vi "Labial Pressure Marker.vi"(6 "Upper SPL":dbl, 8 "Error In":errorcluster, 9 "File Path":path, 10 "Pressure/Audio":dynamicdata(graph)) -> (0 "Error Out":errorcluster, 1 "File Path Indicator":path, 3 "Pressure Array":dbl[](array[numeric]))   [LabVIEW 2020, in "AnalysisSupport.lvlib"]
uses:
  AnalysisSupport.lvlib
  <vilib>/Utility/miscctls.llb/LVCursorListTypeDef.ctl
  <vilib>/Waveform/WDTOps.llb/WDT Get XY Value DBL.vi
panel:
  in  "Undo Button":bool
  out "Upper SPL Bound":dbl
  out "SPL":dbl
  out "Subset":dynamicdata(graph)
  out "Pressure":dynamicdata(graph)
  out "Interruptions Marked":i32
  out "Pressure":dbl
  in  "Done":bool
  in  "Add":bool
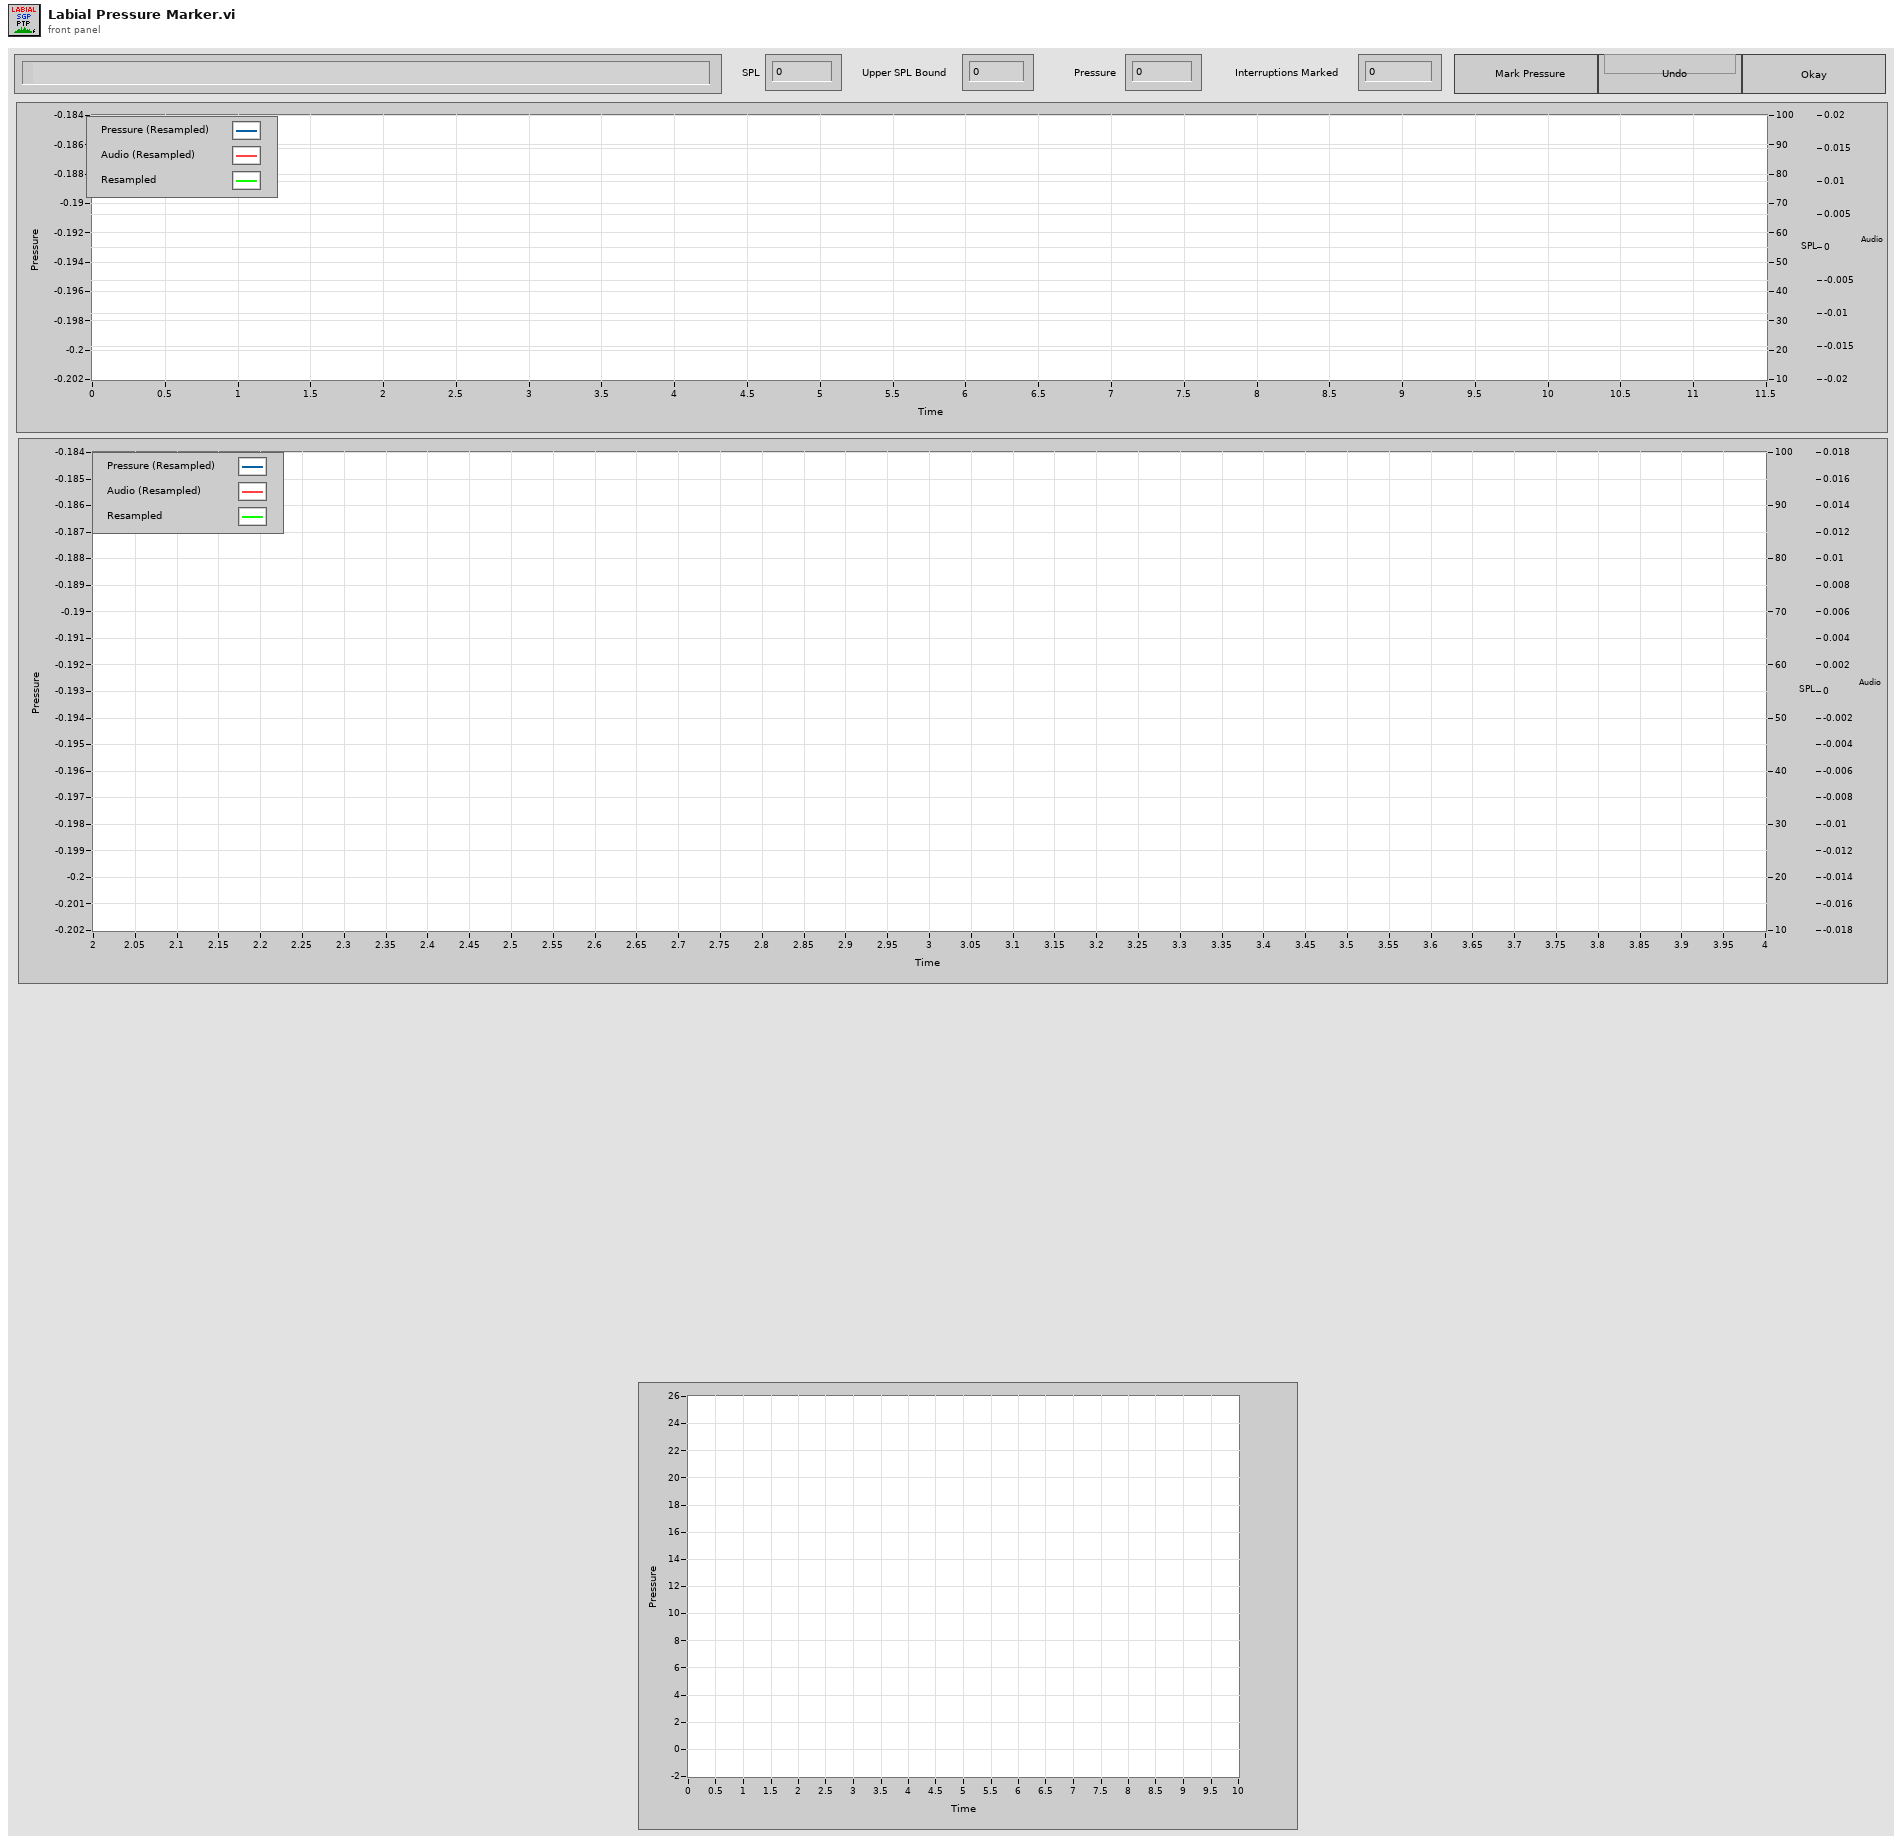
[diagram p1: front panel]
types:
  T1 = typedef "LVCursorListTypeDef.ctl" = cluster{"Name":string, "Color":u32, "Style":u8, "Point Style":u8, "Name Visible":bool, "Allow Drag":bool, "Cursor Mode":u32, "Plot":i32, "Index":i32, "Position":cluster{"X":dbl, "Y":dbl}, "X Scale":u32, "Y Scale":u32, "Watch Plots":i32[], "Watch All Plots":bool, "Plot Area":i32, "Label Offset":cluster{"X":dbl, "Y":dbl}}[]
  T2 = cluster{"Cursor List[0]":cluster{"Name":string, "Color":u32, "Style":u8, "Point Style":u8, "Name Visible":bool, "Allow Drag":bool, "Cursor Mode":u32, "Plot":i32, "Index":i32, "Position":cluster{"X":dbl, "Y":dbl}, "X Scale":u32, "Y Scale":u32, "Watch Plots":i32[], "Watch All Plots":bool, "Plot Area":i32, "Label Offset":cluster{"X":dbl, "Y":dbl}}, "Cursor List[1]":cluster{"Name":string, "Color":u32, "Style":u8, "Point Style":u8, "Name Visible":bool, "Allow Drag":bool, "Cursor Mode":u32, "Plot":i32, "Index":i32, "Position":cluster{"X":dbl, "Y":dbl}, "X Scale":u32, "Y Scale":u32, "Watch Plots":i32[], "Watch All Plots":bool, "Plot Area":i32, "Label Offset":cluster{"X":dbl, "Y":dbl}}, "Cursor List[2]":cluster{"Name":string, "Color":u32, "Style":u8, "Point Style":u8, "Name Visible":bool, "Allow Drag":bool, "Cursor Mode":u32, "Plot":i32, "Index":i32, "Position":cluster{"X":dbl, "Y":dbl}, "X Scale":u32, "Y Scale":u32, "Watch Plots":i32[], "Watch All Plots":bool, "Plot Area":i32, "Label Offset":cluster{"X":dbl, "Y":dbl}}, "Cursor List[3]":cluster{"Name":string, "Color":u32, "Style":u8, "Point Style":u8, "Name Visible":bool, "Allow Drag":bool, "Cursor Mode":u32, "Plot":i32, "Index":i32, "Position":cluster{"X":dbl, "Y":dbl}, "X Scale":u32, "Y Scale":u32, "Watch Plots":i32[], "Watch All Plots":bool, "Plot Area":i32, "Label Offset":cluster{"X":dbl, "Y":dbl}}, "Cursor List[4]":cluster{"Name":string, "Color":u32, "Style":u8, "Point Style":u8, "Name Visible":bool, "Allow Drag":bool, "Cursor Mode":u32, "Plot":i32, "Index":i32, "Position":cluster{"X":dbl, "Y":dbl}, "X Scale":u32, "Y Scale":u32, "Watch Plots":i32[], "Watch All Plots":bool, "Plot Area":i32, "Label Offset":cluster{"X":dbl, "Y":dbl}}, "Cursor List[5]":cluster{"Name":string, "Color":u32, "Style":u8, "Point Style":u8, "Name Visible":bool, "Allow Drag":bool, "Cursor Mode":u32, "Plot":i32, "Index":i32, "Position":cluster{"X":dbl, "Y":dbl}, "X Scale":u32, "Y Scale":u32, "Watch Plots":i32[], "Watch All Plots":bool, "Plot Area":i32, "Label Offset":cluster{"X":dbl, "Y":dbl}}, "Cursor List[6]":cluster{"Name":string, "Color":u32, "Style":u8, "Point Style":u8, "Name Visible":bool, "Allow Drag":bool, "Cursor Mode":u32, "Plot":i32, "Index":i32, "Position":cluster{"X":dbl, "Y":dbl}, "X Scale":u32, "Y Scale":u32, "Watch Plots":i32[], "Watch All Plots":bool, "Plot Area":i32, "Label Offset":cluster{"X":dbl, "Y":dbl}}, "Cursor List[7]":cluster{"Name":string, "Color":u32, "Style":u8, "Point Style":u8, "Name Visible":bool, "Allow Drag":bool, "Cursor Mode":u32, "Plot":i32, "Index":i32, "Position":cluster{"X":dbl, "Y":dbl}, "X Scale":u32, "Y Scale":u32, "Watch Plots":i32[], "Watch All Plots":bool, "Plot Area":i32, "Label Offset":cluster{"X":dbl, "Y":dbl}}, "Cursor List[8]":cluster{"Name":string, "Color":u32, "Style":u8, "Point Style":u8, "Name Visible":bool, "Allow Drag":bool, "Cursor Mode":u32, "Plot":i32, "Index":i32, "Position":cluster{"X":dbl, "Y":dbl}, "X Scale":u32, "Y Scale":u32, "Watch Plots":i32[], "Watch All Plots":bool, "Plot Area":i32, "Label Offset":cluster{"X":dbl, "Y":dbl}}}
  T3 = cluster{"Name":string, "Color":u32, "Style":u8, "Point Style":u8, "Name Visible":bool, "Allow Drag":bool, "Cursor Mode":u32, "Plot":i32, "Index":i32, "Position":cluster{"X":dbl, "Y":dbl}, "X Scale":u32, "Y Scale":u32, "Watch Plots":i32[], "Watch All Plots":bool, "Plot Area":i32, "Label Offset":cluster{"X":dbl, "Y":dbl}}[]
  T4 = cluster{"CrsrList[0]":cluster{"Name":string, "Color":u32, "Style":u8, "Point Style":u8, "Name Visible":bool, "Allow Drag":bool, "Cursor Mode":u32, "Plot":i32, "Index":i32, "Position":cluster{"X":dbl, "Y":dbl}, "X Scale":u32, "Y Scale":u32, "Watch Plots":i32[], "Watch All Plots":bool, "Plot Area":i32, "Label Offset":cluster{"X":dbl, "Y":dbl}}, "CrsrList[1]":cluster{"Name":string, "Color":u32, "Style":u8, "Point Style":u8, "Name Visible":bool, "Allow Drag":bool, "Cursor Mode":u32, "Plot":i32, "Index":i32, "Position":cluster{"X":dbl, "Y":dbl}, "X Scale":u32, "Y Scale":u32, "Watch Plots":i32[], "Watch All Plots":bool, "Plot Area":i32, "Label Offset":cluster{"X":dbl, "Y":dbl}}, "CrsrList[2]":cluster{"Name":string, "Color":u32, "Style":u8, "Point Style":u8, "Name Visible":bool, "Allow Drag":bool, "Cursor Mode":u32, "Plot":i32, "Index":i32, "Position":cluster{"X":dbl, "Y":dbl}, "X Scale":u32, "Y Scale":u32, "Watch Plots":i32[], "Watch All Plots":bool, "Plot Area":i32, "Label Offset":cluster{"X":dbl, "Y":dbl}}, "CrsrList[3]":cluster{"Name":string, "Color":u32, "Style":u8, "Point Style":u8, "Name Visible":bool, "Allow Drag":bool, "Cursor Mode":u32, "Plot":i32, "Index":i32, "Position":cluster{"X":dbl, "Y":dbl}, "X Scale":u32, "Y Scale":u32, "Watch Plots":i32[], "Watch All Plots":bool, "Plot Area":i32, "Label Offset":cluster{"X":dbl, "Y":dbl}}, "CrsrList[4]":cluster{"Name":string, "Color":u32, "Style":u8, "Point Style":u8, "Name Visible":bool, "Allow Drag":bool, "Cursor Mode":u32, "Plot":i32, "Index":i32, "Position":cluster{"X":dbl, "Y":dbl}, "X Scale":u32, "Y Scale":u32, "Watch Plots":i32[], "Watch All Plots":bool, "Plot Area":i32, "Label Offset":cluster{"X":dbl, "Y":dbl}}, "CrsrList[5]":cluster{"Name":string, "Color":u32, "Style":u8, "Point Style":u8, "Name Visible":bool, "Allow Drag":bool, "Cursor Mode":u32, "Plot":i32, "Index":i32, "Position":cluster{"X":dbl, "Y":dbl}, "X Scale":u32, "Y Scale":u32, "Watch Plots":i32[], "Watch All Plots":bool, "Plot Area":i32, "Label Offset":cluster{"X":dbl, "Y":dbl}}, "CrsrList[6]":cluster{"Name":string, "Color":u32, "Style":u8, "Point Style":u8, "Name Visible":bool, "Allow Drag":bool, "Cursor Mode":u32, "Plot":i32, "Index":i32, "Position":cluster{"X":dbl, "Y":dbl}, "X Scale":u32, "Y Scale":u32, "Watch Plots":i32[], "Watch All Plots":bool, "Plot Area":i32, "Label Offset":cluster{"X":dbl, "Y":dbl}}, "CrsrList[7]":cluster{"Name":string, "Color":u32, "Style":u8, "Point Style":u8, "Name Visible":bool, "Allow Drag":bool, "Cursor Mode":u32, "Plot":i32, "Index":i32, "Position":cluster{"X":dbl, "Y":dbl}, "X Scale":u32, "Y Scale":u32, "Watch Plots":i32[], "Watch All Plots":bool, "Plot Area":i32, "Label Offset":cluster{"X":dbl, "Y":dbl}}, "CrsrList[8]":cluster{"Name":string, "Color":u32, "Style":u8, "Point Style":u8, "Name Visible":bool, "Allow Drag":bool, "Cursor Mode":u32, "Plot":i32, "Index":i32, "Position":cluster{"X":dbl, "Y":dbl}, "X Scale":u32, "Y Scale":u32, "Watch Plots":i32[], "Watch All Plots":bool, "Plot Area":i32, "Label Offset":cluster{"X":dbl, "Y":dbl}}}
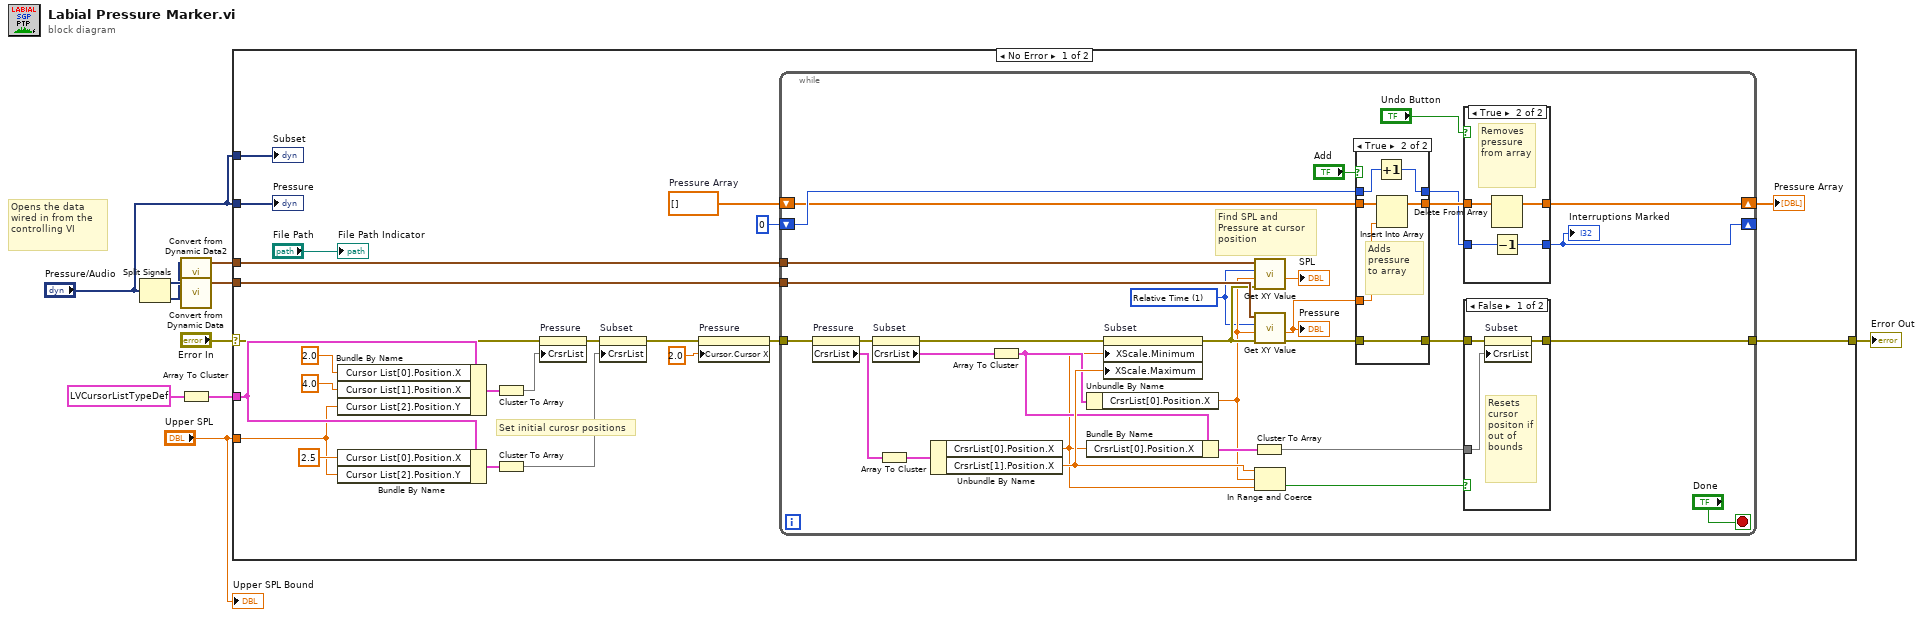
[diagram p0: block diagram]
diagram:
  # "Opens the data wired in from the controlling VI"
  n1 = Split Signals("Pressure/Audio") -> (w4:dynamicdata, w2:dynamicdata)  [unwired: 3 in, 1 out]
  n2 = call "Convert from Dynamic Data2"("Dynamic Data Type"=w2) -> ("Waveform"=w3:waveform(dbl))  [unwired: 3 in]
  n3 = call "Convert from Dynamic Data"("Dynamic Data Type"=w4) -> ("Waveform"=w8:waveform(dbl))  [unwired: 3 in]
  n4 = Array To Cluster(array=T1 [{"Name"="L", "Color"=9843450, "Style"=2, "Point Style"=1, "Name Visible"=FALSE, "Allow Drag"=TRUE, "Cursor Mode"=0, "Plot"=0, "Index"=0, "Position"={"X"=3.0, "Y"=0.0}, "X Scale"=0, "Y Scale"=0, "Watch Plots"=[], "Watch All Plots"=FALSE, "Plot Area"=0, "Label Offset"={"X"=0.0, "Y"=0.0}}, {"Name"="R", "Color"=681210, "Style"=2, "Point Style"=1, "Name Visible"=FALSE, "Allow Drag"=TRUE, "Cursor Mode"=0, "Plot"=0, "Index"=0, "Position"={"X"=-5.0, "Y"=0.0}, "X Scale"=0, "Y Scale"=0, "Watch Plots"=[], "Watch All Plots"=FALSE, "Plot Area"=0, "Label Offset"={"X"=0.0, "Y"=0.0}}, {"Name"="SPL", "Color"=0, "Style"=6, "Point Style"=0, "Name Visible"=FALSE, "Allow Drag"=FALSE, "Cursor Mode"=0, "Plot"=0, "Index"=0, "Position"={"X"=0.0, "Y"=0.0}, "X Scale"=0, "Y Scale"=2, "Watch Plots"=[], "Watch All Plots"=FALSE, "Plot Area"=0, "Label Offset"={"X"=0.0, "Y"=0.0}}] ("Cursor List")) -> (cluster=w6:T2)
  n5 = case shown="No Error" "Error In" {
    selector: "Error In" -> [w14 w84]
    tunnel: [w32 w84] -> w10
    tunnel: "Pressure/Audio" -> [w27 _]
    tunnel: "Pressure/Audio" -> [w29 _]
    tunnel: w8 -> [w28 _]
    tunnel: w6 -> [w18 _]
    tunnel: w3 -> [w12 _]
    tunnel: "Upper SPL" -> [w11 _]
    frame No Error {
      w25 = dbl[] []  # Pressure Array
      # "Set initial curosr positions"
      n6 = Bundle By Name(cluster=w18, "Cursor List[0].Position.X"=2.0, "Cursor List[1].Position.X"=4.0, "Cursor List[2].Position.Y"=w11) -> (w21:T2)
      n7 = Bundle By Name(cluster=w18, "Cursor List[0].Position.X"=2.5, "Cursor List[2].Position.Y"=w11) -> (w16:T2)
      n8 = Cluster To Array(cluster=w21) -> (array=w22:T3)
      n9 = Cluster To Array(cluster=w16) -> (array=w15:T3)
      n10 = property on="Pressure" class="WFGraph (strict)"(error in=w14, "CrsrList"=w22) -> (error out=w23:errorcluster)  [unwired: 1 in, 1 out]
      n11 = property on="Subset" class="WFGraph (strict)"(error in=w23, "CrsrList"=w15) -> (error out=w13:errorcluster)  [unwired: 1 in, 1 out]
      n12 = property on="Pressure" class="WFGraph (strict)"(error in=w13, "Cursor.Cursor X"=2.0 ("Cursor.Cursor Position:Cursor X")) -> (error out=w30:errorcluster)  [unwired: 1 in, 1 out]
      n13 = while {
        tunnel: [w52] -> w32
        tunnel: w30 -> [w44]
        tunnel: w28 -> [w64]
        shift-right: [w35] -> _
        shift-left: 0 -> [w62]
        shift-right: [w36] -> w24
        shift-left: w25 -> [w58]
        tunnel: w12 -> [w41]
        stop <- "Done" stop-if-true
        w40 = u16 1 items=["Samples", "Relative Time"] ("Y position format")
        # "Find SPL and Pressure at cursor position"
        n14 = property on="Pressure" class="WFGraph (strict)"(error in=w44) -> (error out=w57:errorcluster, "CrsrList"=w54:T1)  [unwired: 1 in, 1 out]
        n15 = property on="Subset" class="WFGraph (strict)"(error in=w57) -> (error out=w56:errorcluster, "CrsrList"=w53:T1)  [unwired: 1 in, 1 out]
        n16 = Array To Cluster(array=w54) -> (cluster=w55:T4)
        n17 = Unbundle By Name(w55) -> ("CrsrList[0].Position.X"=w45:dbl, "CrsrList[1].Position.X"=w49:dbl)
        n18 = Array To Cluster(array=w53) -> (cluster=w46:T4)
        n19 = Unbundle By Name(w46) -> ("CrsrList[0].Position.X"=w42:dbl)
        n20 = Bundle By Name(cluster=w46, "CrsrList[0].Position.X"=w45) -> (w47:T4)
        n21 = property on="Subset" class="WFGraph (strict)"(error in=w56, "XScale.Minimum"=w45, "XScale.Maximum"=w49) -> (error out=w43:errorcluster)  [unwired: 1 in, 1 out]
        n22 = Cluster To Array(cluster=w47) -> (array=w48:T3)
        n23 = call-poly <vilib>:"Get XY Value.vi"("error in (no error)"=w43, "Y position"=w42, "Y position format"=w40, "waveform in"=w41) -> ("Y value"=→"SPL":dbl)  [unwired: 3 in, 4 out]
        n24 = call-poly <vilib>:"Get XY Value.vi"("error in (no error)"=w43, "Y position"=w42, "Y position format"=w40, "waveform in"=w64) -> ("error out"=w63:errorcluster, "Y value"=w59:dbl)  [unwired: 3 in, 3 out]
        "Pressure" <- w59
        n25 = In Range and Coerce(upper limit=w49, x=w42, lower limit=w45) -> (In Range?=w50:bool)  [unwired: 1 out]
        n26 = case shown="True" "Add" {
          tunnel: w63 -> [w77 w83]
          tunnel: [w77 w83] -> w51
          tunnel: w62 -> [w76 w82]
          tunnel: [w76 w81] -> w37
          tunnel: w59 -> [_ w78]
          tunnel: w58 -> [w75 w80]
          tunnel: [w75 w79] -> w38
          frame False {
          }
          frame True {
            # "Adds pressure to array"
            n27 = Increment(x=w82) -> (x+1=w81:i32)
            n28 = Insert Into Array(array=w80, new element=w78) -> (w79:dbl[])  [unwired: 1 in]
          }
        }
        n29 = case shown="True" "Undo Button" {
          tunnel: w38 -> [w65 w69]
          tunnel: w37 -> [w66 w67]
          tunnel: [w66 w70] -> w35
          tunnel: [w65 w68] -> w36
          frame False {
          }
          frame True {
            # "Removes pressure from array"
            n30 = Delete From Array(array=w69) -> (array with subset deleted=w68:dbl[])  [unwired: 2 in, 1 out]
            n31 = Decrement(x=w67) -> (x-1=w70:i32)
          }
        }
        "Interruptions Marked" <- w35
        n32 = case shown="False" w50 {
          tunnel: [w73 w74] -> w52
          tunnel: w51 -> [w72 w74]
          tunnel: w48 -> [w71 _]
          frame False {
            # "Resets cursor positon if out of bounds"
            n33 = property on="Subset" class="WFGraph (strict)"(error in=w72, "CrsrList"=w71) -> (error out=w73:errorcluster)  [unwired: 1 in, 1 out]
          }
          frame True {
          }
        }
      }
      "Pressure Array" <- w24
      "File Path Indicator" <- "File Path"
      "Subset" <- w29
      "Pressure" <- w27
    }
    frame Error {
    }
  }
  "Error Out" <- w10
  "Upper SPL Bound" <- "Upper SPL"
